vi "host.vi"() -> ()   [LabVIEW 2020]
uses:
  <vilib>/rvi/interface/RandomDataEmulation/nirviRandomDataOpen.vi
  <vilib>/rvi/interface/common/niFpgaCacheSessionInfoDynamic.vi
  <vilib>/Utility/error.llb/Error Cluster From Error Code.vi
  <vilib>/rvi/interface/common/niFpgaWaitOnOcc.vi
  <vilib>/rvi/errors/niLvFpgaAdjustHostInterfaceError.vi
  <vilib>/FPGAPlugInAG/Dynamic/niLvFpga_Run_Dynamic.vi
  <vilib>/FPGAPlugInAG/Dynamic/niLvFpga_Close_Dynamic.vi
  <vilib>/rvi/interface/nirviOpenFPGA/nirviOpenFPGA.xnode
  FFT.vi
  <vilib>/rvi/interface/nirviMethod/nirviMethod.xnode
  <vilib>/rvi/interface/nirviCloseFPGA/nirviCloseFPGA.xnode
  <vilib>/rvi/errors/niLvFpgaMergeErrorWithErrorCode.vi
  <vilib>/Analysis/NI_AALPro.lvlib
  <vilib>/FPGAPlugInAG/Dynamic/niLvFpga_ReadFifo_Dynamic.vi
  <vilib>/FPGAPlugInAG/Dynamic/niLvFpga_ConfigureFifo_Dynamic.vi
  <vilib>/FPGAPlugInAG/Dynamic/niLvFpga_StartFifo_Dynamic.vi
  <vilib>/FPGAPlugInAG/Dynamic/niLvFpga_WriteFifo_Dynamic.vi
panel:
  out "array faul":dbl[](graph)
  out "array faul":i32
  out "array faul 2":fxp<+/-,32,16>[](array[numeric])
  out "freq index":dbl[](array[numeric])
  out "phase 2 index":dbl[](graph)
  out "phase 2 size":i32
  out "mag 2 index":dbl[](graph)
  out "mag 2 size":i32
  out "phase 2":fxp<+/-,32,15>[](array[numeric])
  out "mag 2":fxp<+/-,32,15>[](array[numeric])
  out "frequency index":dbl[](graph)
  out "frequency size":i32
  out "freq":fxp<+/-,32,15>[](array[numeric])
  out "magnitude":dbl[](graph)
  out "phase":dbl[](graph)
  out "phase size":i32
  out "mag size":i32
  out "phase 3":fxp<+/-,32,15>[](array[numeric])
  out "magnitude 2":fxp<+/-,32,15>[](array[numeric])
  out "Actual Depth":u32
  out "host to target":u32
  out "signal_target_to_host_fixed size(s)":i32
  out "target to host 1":u32
  out "signal target to host":dbl[][](graph)
  out "signal_target_to_host_fixed":fxp<+/-,24,7>[](array[numeric])
  out "Array 2":fxp<+/-,24,7>[](array[numeric])
  out "detrend acc":dbl[](graph)
  out "samples":i32
  out "input signal":T1(graph)
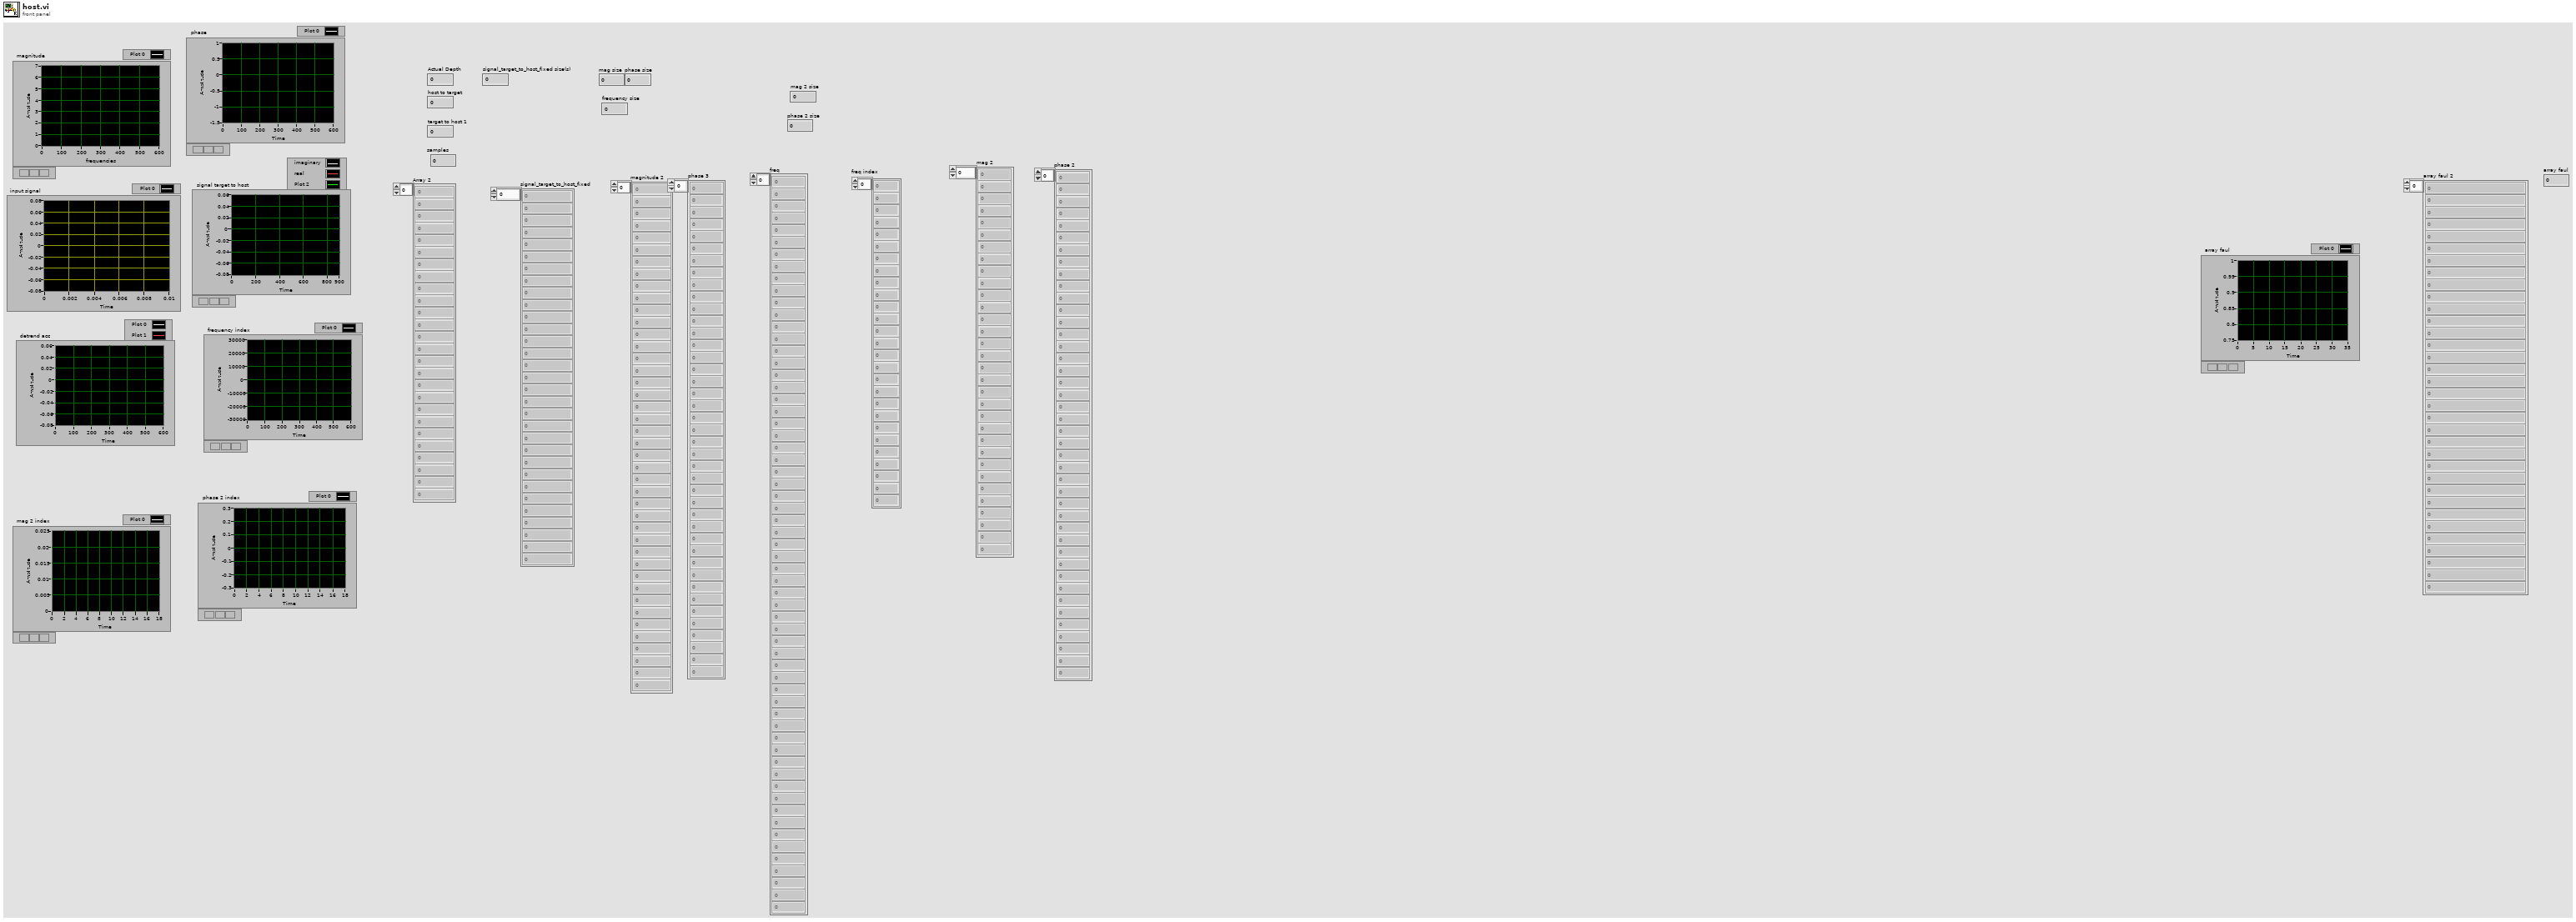
[diagram p1: front panel]
types:
  T1 = cluster{"array type (2D Dbl)":dbl[], "array type (2D Dbl)":dbl[]}
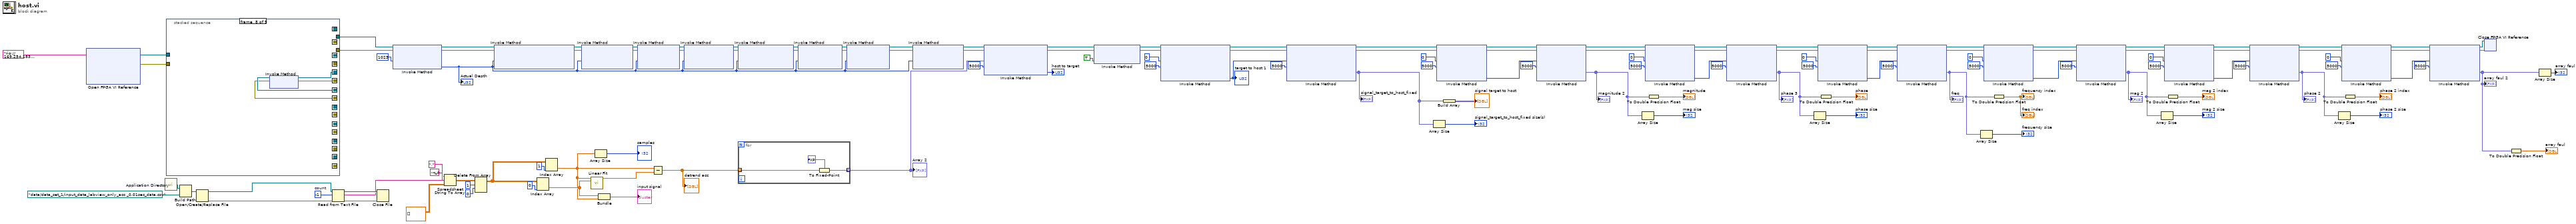
[diagram p0: block diagram]
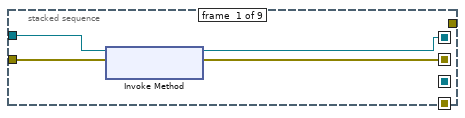
[diagram p2: hidden frame]
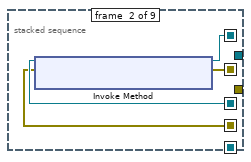
[diagram p3: hidden frame]
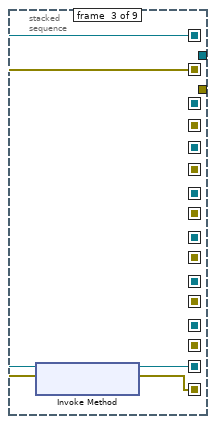
[diagram p4: hidden frame]
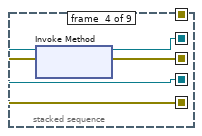
[diagram p5: hidden frame]
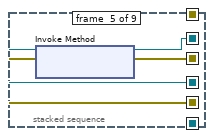
[diagram p6: hidden frame]
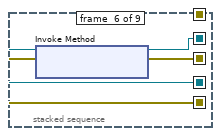
[diagram p7: hidden frame]
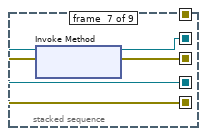
[diagram p8: hidden frame]
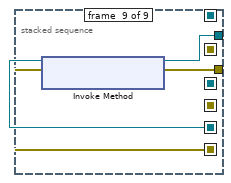
[diagram p9: hidden frame]
diagram:
  w125 = -1  # count
  n1 = xnode "Open FPGA VI Reference"("resource name"=tag "rio://169.254.183.73/RIO0") -> ("FPGA VI Reference Out"=w95:refnum<k20>, "error out"=w94:errorcluster)  [unwired: 1 in]
  n2 = call <vilib>:"Application Directory.vi"() -> ("Application Directory"=w129:path)
  n3 = stacked-sequence {
    seq-local: [w136 _ _ _ _ _ _ _ _] -> [_ w142 _ _ _ _ _ _ _]
    seq-local: [w135 _ _ _ _ _ _ _ _] -> [_ w141 _ _ _ _ _ _ _]
    seq-local: [_ w140 _ _ _ _ _ _ _] -> [_ _ w146 _ _ _ _ _ _]
    seq-local: [_ w139 _ _ _ _ _ _ _] -> [_ _ w145 _ _ _ _ _ _]
    seq-local: [_ _ w144 _ _ _ _ _ _] -> [_ _ _ w150 _ _ _ _ _]
    seq-local: [_ _ w143 _ _ _ _ _ _] -> [_ _ _ w149 _ _ _ _ _]
    seq-local: [_ _ _ w148 _ _ _ _ _] -> [_ _ _ _ w154 _ _ _ _]
    seq-local: [_ _ _ w147 _ _ _ _ _] -> [_ _ _ _ w153 _ _ _ _]
    seq-local: [_ _ _ _ w152 _ _ _ _] -> [_ _ _ _ _ w158 _ _ _]
    seq-local: [_ _ _ _ w151 _ _ _ _] -> [_ _ _ _ _ w157 _ _ _]
    seq-local: [_ _ _ _ _ w156 _ _ _] -> [_ _ _ _ _ _ w162 _ _]
    seq-local: [_ _ _ _ _ w155 _ _ _] -> [_ _ _ _ _ _ w161 _ _]
    seq-local: [_ _ _ _ _ _ w160 _ _] -> [_ _ _ _ _ _ _ w165 _]
    seq-local: [_ _ _ _ _ _ w159 _ _] -> [_ _ _ _ _ _ _ w166 _]
    seq-local: [_ _ _ _ _ _ _ w164 _] -> [_ _ _ _ _ _ _ _ w170]
    seq-local: [_ _ _ _ _ _ _ w163 _] -> [_ _ _ _ _ _ _ _ w169]
    tunnel: w95 -> [w138 _ _ _ _ _ _ _ _]
    tunnel: w94 -> [w137 _ _ _ _ _ _ _ _]
    tunnel: [_ _ _ _ _ _ _ _ w168] -> w18
    tunnel: [_ _ _ _ _ _ _ _ w167] -> w17
    frame #0 {
      n4 = xnode "Invoke Method"("FPGA VI Reference In"=w138, "error in"=w137) -> ("FPGA VI Reference Out"=w136:refnum<k20>, "error out"=w135:errorcluster)
    }
    frame #1 {
      n5 = xnode "Invoke Method"("FPGA VI Reference In"=w142, "error in"=w141) -> ("FPGA VI Reference Out"=w140:refnum<k20>, "error out"=w139:errorcluster)
    }
    frame #2 {
      n6 = xnode "Invoke Method"("FPGA VI Reference In"=w146, "error in"=w145) -> ("FPGA VI Reference Out"=w144:refnum<k20>, "error out"=w143:errorcluster)
    }
    frame #3 {
      n7 = xnode "Invoke Method"("FPGA VI Reference In"=w150, "error in"=w149) -> ("FPGA VI Reference Out"=w148:refnum<k20>, "error out"=w147:errorcluster)
    }
    frame #4 {
      n8 = xnode "Invoke Method"("FPGA VI Reference In"=w154, "error in"=w153) -> ("FPGA VI Reference Out"=w152:refnum<k20>, "error out"=w151:errorcluster)
    }
    frame #5 {
      n9 = xnode "Invoke Method"("FPGA VI Reference In"=w158, "error in"=w157) -> ("FPGA VI Reference Out"=w156:refnum<k20>, "error out"=w155:errorcluster)
    }
    frame #6 {
      n10 = xnode "Invoke Method"("FPGA VI Reference In"=w162, "error in"=w161) -> ("FPGA VI Reference Out"=w159:refnum<k20>, "error out"=w160:errorcluster)
    }
    frame #7 {
      n11 = xnode "Invoke Method"("FPGA VI Reference In"=w166, "error in"=w165) -> ("FPGA VI Reference Out"=w164:refnum<k20>, "error out"=w163:errorcluster)
    }
    frame #8 {
      n12 = xnode "Invoke Method"("FPGA VI Reference In"=w170, "error in"=w169) -> ("FPGA VI Reference Out"=w168:refnum<k20>, "error out"=w167:errorcluster)
    }
  }
  n13 = Build Path(base path=w129, name or relative path=path "data/data_set_1/input_data_labview_only_acc _0.01sec_data.csv" ("default name")) -> (appended path=w128:path)
  n14 = Open/Create/Replace File(file path (use dialog)=w128) -> (refnum out=w133:refnum<file>, error out=w134:errorcluster)  [unwired: 5 in, 1 out]
  n15 = Read from Text File(file (use dialog)=w133, count=w125, error in=w134) -> (refnum out=w132:refnum<file>, text=w130:string, error out=w131:errorcluster)  [unwired: 1 in, 1 out]
  n16 = Close File(refnum=w132, error in=w131) -> ()  [unwired: 2 out]
  n17 = xnode "Invoke Method"("FPGA VI Reference In"=w18, "error in"=w17, "Requested Depth"=u32 1023) -> ("FPGA VI Reference Out"=w93:refnum<k20>, "error out"=w92:errorcluster, "Actual Depth"=w23:u32)
  "Actual Depth" <- w23
  n18 = Spreadsheet String To Array(delimiter (Tab)=",", format string="%f", spreadsheet string=w130, array type (2D Dbl)=dbl[][] []) -> (array=w122:dbl[][])
  n19 = Delete From Array(array=w122, length=1, index (row)=0) -> (array with subset deleted=w117:dbl[][])  [unwired: 1 in, 1 out]
  n20 = xnode "Invoke Method"("FPGA VI Reference In"=w93, "error in"=w92, "Requested Depth"=w23) -> ("FPGA VI Reference Out"=w91:refnum<k20>, "error out"=w90:errorcluster)  [unwired: 1 out]
  n21 = Index Array(array=w117, index (col)=0 ("disabled index (col)")) -> (element=w15:dbl[])  [unwired: 1 in]
  n22 = Index Array(array=w117, index (col)=1 ("disabled index (col)")) -> (element=w14:dbl[])  [unwired: 1 in]
  n23 = xnode "Invoke Method"("FPGA VI Reference In"=w91, "error in"=w90, "Requested Depth"=w23) -> ("FPGA VI Reference Out"=w89:refnum<k20>, "error out"=w88:errorcluster)  [unwired: 1 out]
  n24 = call <vilib>:"Linear Fit.vi"("Y"=w14, "X"=w15) -> ("Best Linear Fit"=w16:dbl[])  [unwired: 9 in, 4 out]
  n25 = Array Size(array=w14) -> (size(s)=→"samples":i32)
  n26 = Bundle("array type (2D Dbl)"=w15, "array type (2D Dbl)"=w14) -> (→"input signal":T1)  [unwired: 1 in]
  n27 = xnode "Invoke Method"("FPGA VI Reference In"=w89, "error in"=w88, "Requested Depth"=w23) -> ("FPGA VI Reference Out"=w55:refnum<k20>, "error out"=w54:errorcluster)  [unwired: 1 out]
  n28 = Subtract(x=w14, y=w16) -> (x-y=w109:dbl[])
  "detrend acc" <- w109
  n29 = xnode "Invoke Method"("FPGA VI Reference In"=w55, "error in"=w54, "Requested Depth"=w23) -> ("FPGA VI Reference Out"=w31:refnum<k20>, "error out"=w30:errorcluster)  [unwired: 1 out]
  n30 = xnode "Invoke Method"("FPGA VI Reference In"=w31, "error in"=w30, "Requested Depth"=w23) -> ("FPGA VI Reference Out"=w33:refnum<k20>, "error out"=w32:errorcluster)  [unwired: 1 out]
  n31 = for {
    tunnel: [w172] -> w108 mode=indexing
    tunnel: w109 -> [w171] mode=indexing
    n32 = To Fixed-Point(fixed-point type=fxp<+/-,24,7> 0.0 ("f"), number=w171) -> (fixed-point=w172:fxp<+/-,24,7>)
  }
  "Array 2" <- w108
  n33 = xnode "Invoke Method"("FPGA VI Reference In"=w33, "error in"=w32, "Requested Depth"=w23) -> ("FPGA VI Reference Out"=w25:refnum<k20>, "error out"=w24:errorcluster)  [unwired: 1 out]
  n34 = xnode "Invoke Method"("FPGA VI Reference In"=w25, "error in"=w24, "Requested Depth"=w23) -> ("FPGA VI Reference Out"=w22:refnum<k20>, "error out"=w21:errorcluster)  [unwired: 1 out]
  n35 = xnode "Invoke Method"("FPGA VI Reference In"=w22, "error in"=w21, "Requested Depth"=w23) -> ("FPGA VI Reference Out"=w20:refnum<k20>, "error out"=w19:errorcluster)  [unwired: 1 out]
  n36 = xnode "Invoke Method"("FPGA VI Reference In"=w20, "error in"=w19, "Data"=w108, "Timeout (ms)"=5000) -> ("FPGA VI Reference Out"=w114:refnum<k20>, "error out"=w113:errorcluster, "Empty Elements Remaining"=→"host to target":u32)
  n37 = xnode "Invoke Method"("FPGA VI Reference In"=w114, "error in"=w113, "Wait Until Done (F)"=TRUE) -> ("FPGA VI Reference Out"=w99:refnum<k20>, "error out"=w98:errorcluster)
  n38 = xnode "Invoke Method"("FPGA VI Reference In"=w99, "error in"=w98, "Number of Elements"=u32 0, "Timeout (ms)"=5000) -> ("FPGA VI Reference Out"=w107:refnum<k20>, "error out"=w106:errorcluster, "Elements Remaining"=w105:u32)  [unwired: 1 out]
  "target to host 1" <- w105
  n39 = xnode "Invoke Method"("FPGA VI Reference In"=w107, "error in"=w106, "Number of Elements"=w105, "Timeout (ms)"=5000) -> ("FPGA VI Reference Out"=w70:refnum<k20>, "error out"=w69:errorcluster, "Data"=w101:fxp<+/-,24,7>[])  [unwired: 1 out]
  "signal_target_to_host_fixed" <- w101
  n40 = Array Size(array=w101) -> (size(s)=→"signal_target_to_host_fixed size(s)":i32)
  n41 = xnode "Invoke Method"("FPGA VI Reference In"=w70, "error in"=w69, "Number of Elements"=u32 0, "Timeout (ms)"=5000) -> ("FPGA VI Reference Out"=w84:refnum<k20>, "error out"=w83:errorcluster, "Elements Remaining"=w78:u32)  [unwired: 1 out]
  n42 = Build Array(w101) -> (→"signal target to host":fxp<+/-,24,7>[][])
  n43 = xnode "Invoke Method"("FPGA VI Reference In"=w84, "error in"=w83, "Number of Elements"=w78, "Timeout (ms)"=5000) -> ("FPGA VI Reference Out"=w82:refnum<k20>, "error out"=w81:errorcluster, "Data"=w68:fxp<+/-,32,16>[])  [unwired: 1 out]
  "magnitude 2" <- w68
  n44 = Array Size(array=w68) -> (size(s)=→"mag size":i32)
  n45 = xnode "Invoke Method"("FPGA VI Reference In"=w82, "error in"=w81, "Number of Elements"=u32 0, "Timeout (ms)"=5000) -> ("FPGA VI Reference Out"=w80:refnum<k20>, "error out"=w79:errorcluster, "Elements Remaining"=w74:u32)  [unwired: 1 out]
  n46 = To Double Precision Float(number=w68) -> (double precision float=→"magnitude":dbl[])
  n47 = xnode "Invoke Method"("FPGA VI Reference In"=w80, "error in"=w79, "Number of Elements"=w74, "Timeout (ms)"=5000) -> ("FPGA VI Reference Out"=w57:refnum<k20>, "error out"=w56:errorcluster, "Data"=w67:fxp<+/-,16,2>[])  [unwired: 1 out]
  "phase 3" <- w67
  n48 = Array Size(array=w67) -> (size(s)=→"phase size":i32)
  n49 = xnode "Invoke Method"("FPGA VI Reference In"=w57, "error in"=w56, "Number of Elements"=u32 0, "Timeout (ms)"=5000) -> ("FPGA VI Reference Out"=w66:refnum<k20>, "error out"=w65:errorcluster, "Elements Remaining"=w62:u32)  [unwired: 1 out]
  n50 = To Double Precision Float(number=w67) -> (double precision float=→"phase":dbl[])
  n51 = xnode "Invoke Method"("FPGA VI Reference In"=w66, "error in"=w65, "Number of Elements"=w62, "Timeout (ms)"=5000) -> ("FPGA VI Reference Out"=w41:refnum<k20>, "error out"=w40:errorcluster, "Data"=w59:fxp<+/-,32,16>[])  [unwired: 1 out]
  "freq" <- w59
  n52 = Array Size(array=w59) -> (size(s)=→"frequency size":i32)
  n53 = xnode "Invoke Method"("FPGA VI Reference In"=w41, "error in"=w40, "Number of Elements"=u32 0, "Timeout (ms)"=5000) -> ("FPGA VI Reference Out"=w53:refnum<k20>, "error out"=w52:errorcluster, "Elements Remaining"=w49:u32)  [unwired: 1 out]
  n54 = To Double Precision Float(number=w59) -> (double precision float=→"frequency index" →"freq index":dbl[])
  n55 = xnode "Invoke Method"("FPGA VI Reference In"=w53, "error in"=w52, "Number of Elements"=w49, "Timeout (ms)"=5000) -> ("FPGA VI Reference Out"=w39:refnum<k20>, "error out"=w38:errorcluster, "Data"=w35:fxp<+/-,32,16>[])  [unwired: 1 out]
  "mag 2" <- w35
  n56 = Array Size(array=w35) -> (size(s)=→"mag 2 size":i32)
  n57 = xnode "Invoke Method"("FPGA VI Reference In"=w39, "error in"=w38, "Number of Elements"=u32 0, "Timeout (ms)"=5000) -> ("FPGA VI Reference Out"=w47:refnum<k20>, "error out"=w46:errorcluster, "Elements Remaining"=w43:u32)  [unwired: 1 out]
  n58 = To Double Precision Float(number=w35) -> (double precision float=→"mag 2 index":dbl[])
  n59 = xnode "Invoke Method"("FPGA VI Reference In"=w47, "error in"=w46, "Number of Elements"=w43, "Timeout (ms)"=5000) -> ("FPGA VI Reference Out"=w7:refnum<k20>, "error out"=w6:errorcluster, "Data"=w34:fxp<+/-,32,16>[])  [unwired: 1 out]
  "phase 2" <- w34
  n60 = Array Size(array=w34) -> (size(s)=→"phase 2 size":i32)
  n61 = xnode "Invoke Method"("FPGA VI Reference In"=w7, "error in"=w6, "Number of Elements"=u32 0, "Timeout (ms)"=5000) -> ("FPGA VI Reference Out"=w13:refnum<k20>, "error out"=w12:errorcluster, "Elements Remaining"=w9:u32)  [unwired: 1 out]
  n62 = To Double Precision Float(number=w34) -> (double precision float=→"phase 2 index":dbl[])
  n63 = xnode "Invoke Method"("FPGA VI Reference In"=w13, "error in"=w12, "Number of Elements"=w9, "Timeout (ms)"=5000) -> ("FPGA VI Reference Out"=w5:refnum<k20>, "error out"=w4:errorcluster, "Data"=w1:fxp<+/-,32,2>[])  [unwired: 1 out]
  "array faul 2" <- w1
  n64 = xnode "Close FPGA VI Reference"("FPGA VI Reference In"=w5, "error in"=w4) -> ()  [unwired: 1 out]
  n65 = To Double Precision Float(number=w1) -> (double precision float=→"array faul":dbl[])
  n66 = Array Size(array=w1) -> (size(s)=→"array faul":i32)
